vi "REPORT_DATES_status_number_to_description_and_enum.vi"(11 "status_nmb":string) -> (2 "status_enum":T1, 3 "status_description":string)   [LabVIEW 2019]
uses:
  typedef/REPORT_DATES_statuses.ctl
  _misc/AULocalize/SubVIs/Get Localized Phrase Compact Interface 0D.vi
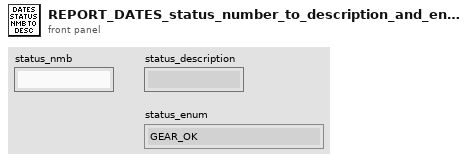
[diagram p1: front panel]
types:
  T1 = typedef "REPORT_DATES_statuses.ctl" = enum16{"GEAR_OK", "GEAR_NOK", "GEAR_interrupted", "GEAR_in_operation", "GEAR_unexpected"}
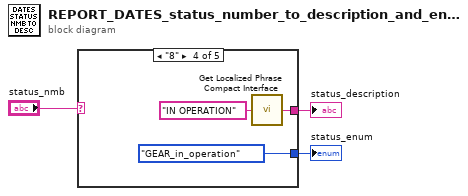
[diagram p0: block diagram]
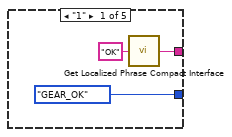
[diagram p2: hidden frame]
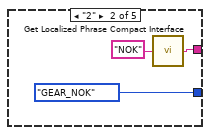
[diagram p3: hidden frame]
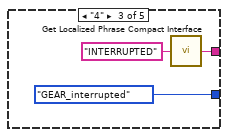
[diagram p4: hidden frame]
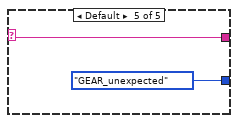
[diagram p5: hidden frame]
diagram:
  n1 = case shown="\"8\"" "status_nmb" {
    selector: "status_nmb" -> [_ _ _ _ w16]
    tunnel: [REPORT_DATES_statuses."GEAR_OK" ("REPORT_DATES_statuses") REPORT_DATES_statuses."GEAR_NOK" ("REPORT_DATES_statuses") REPORT_DATES_statuses."GEAR_interrupted" ("REPORT_DATES_statuses") REPORT_DATES_statuses."GEAR_in_operation" ("REPORT_DATES_statuses") REPORT_DATES_statuses."GEAR_unexpected" ("REPORT_DATES_statuses")] -> w2
    tunnel: [w4 w7 w10 w13 w16] -> w3
    frame "1" {
      n2 = call-poly "Get Localized Phrase Compact Interface.vi"("Key"="OK") -> ("Translated Phrase"=w4:string)
    }
    frame "2" {
      n3 = call-poly "Get Localized Phrase Compact Interface.vi"("Key"="NOK") -> ("Translated Phrase"=w7:string)
    }
    frame "4" {
      n4 = call-poly "Get Localized Phrase Compact Interface.vi"("Key"="INTERRUPTED") -> ("Translated Phrase"=w10:string)
    }
    frame "8" {
      n5 = call-poly "Get Localized Phrase Compact Interface.vi"("Key"="IN OPERATION") -> ("Translated Phrase"=w13:string)
    }
    frame Default {
    }
  }
  "status_description" <- w3
  "status_enum" <- w2
